vi "Close.vi"(8 "error in":errorcluster, 11 "lia rt in":refnum<class "Lock-In Amplifier Example RT.lvclass">) -> (0 "error out":errorcluster, 3 "lia rt out":refnum<class "Lock-In Amplifier Example RT.lvclass">)   [LabVIEW 2017, in "Lock-In Amplifier Example RT.lvclass"]
uses:
  Lock-In Amplifier Example RT.lvclass
  Lock-In Amplifier Example RT.lvclass/Lock-In Amplifier Example RT.ctl
  interface/Interface FPGA/LIA Host Interface FPGA.lvclass
  server/RT FlexRIO Server TCP.lvclass
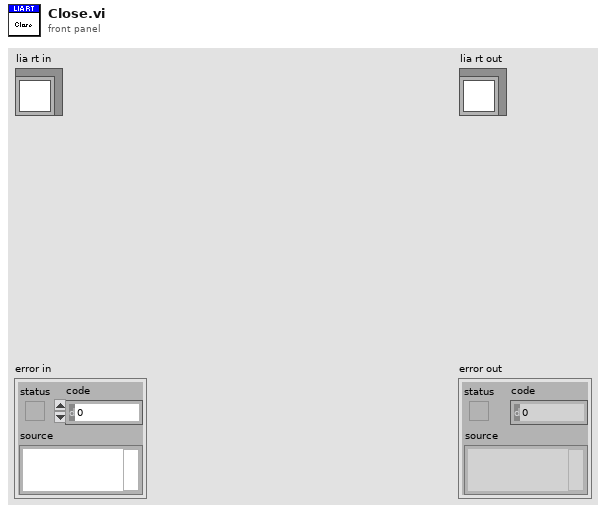
[diagram p1: front panel]
types:
  T1 = typedef "Lock-In Amplifier Example RT.lvclass/session data.ctl" = cluster{"server":refnum<class "RT FlexRIO Server TCP.lvclass">, "fpga interface":refnum<class "LIA Host Interface FPGA.lvclass">}
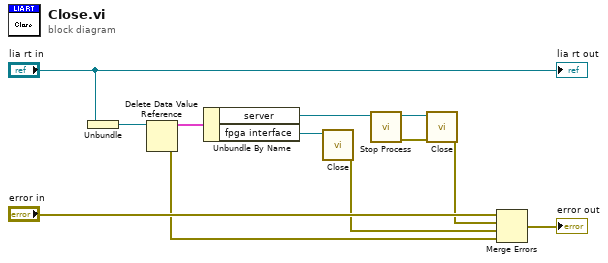
[diagram p0: block diagram]
diagram:
  n1 = Unbundle("lia rt in") -> (w11:refnum<data-value>)
  n2 = Delete Data Value Reference(data value reference=w11) -> (data value=w10:T1, error out=w1:errorcluster)  [unwired: 1 in]
  n3 = Unbundle By Name(w10) -> ("server"=w6:refnum<class "RT FlexRIO Server TCP.lvclass">, "fpga interface"=w4:refnum<class "LIA Host Interface FPGA.lvclass">)
  n4 = call-dynamic "Close.vi"("host in"=w4) -> ("error out"=w2:errorcluster)  [unwired: 9 in, 1 out]
  n5 = call "Stop Process.vi"("tcp server in"=w6) -> ("error out"=w3:errorcluster, "tcp server out"=w5:refnum<class "RT FlexRIO Server TCP.lvclass">)  [unwired: 9 in]
  n6 = call-dynamic "Close.vi"("error in"=w3, "tcp server in"=w5) -> ("error out"=w7:errorcluster)  [unwired: 8 in, 1 out]
  n7 = Merge Errors("error in", w7, w2, w1) -> (→"error out":errorcluster)
  "lia rt out" <- "lia rt in"
